vi "Periodic Tasks[Conflict].vi"(8 "error in":errorcluster) -> ()   [LabVIEW 2019]
doc: "This VI runs in parallel to other tasks. It can contain as many user-defined periodic loops as you need. These can carry out PID or other sorts of timed response."
uses:
  <vilib>/Rock Robotics/WPI/ThirdParty/Phoenix-LabVIEW/Motor Controller/Controls/CTRE_Phoenix_MotorControl_ControlMode.ctl
  <vilib>/Rock Robotics/Network Tables/NT Read Number.vi
  <vilib>/Rock Robotics/WPI/ThirdParty/Phoenix-LabVIEW/Motor Controller/Get/CTRE_Phoenix_MotorController_GetSupplyAndStatorCurrent_Enhanced.vi
  <vilib>/Rock Robotics/WPI/ThirdParty/Phoenix-LabVIEW/Motor Controller/Get/CTRE_Phoenix_MotorController_GetSelectedSensorData.vi
  <vilib>/gmath/NI_Gmath.lvlib
panel:
  out "element":dbl
  in  "PIDF?":bool
  in  "Target RPM":dbl
  out "Rpm":cluster{dbl, "Target RPM":dbl}(graph)
  out "Current":T1(graph)
  in  "PIDF Slot":i32
  in  "I-Zone":dbl
  in  "F":dbl=0.055
  in  "D":dbl
  in  "I":dbl
  in  "P":dbl
  out "Target Dist":dbl
  out "Outtake Sensor":bool
  out "Intake Sensor":bool
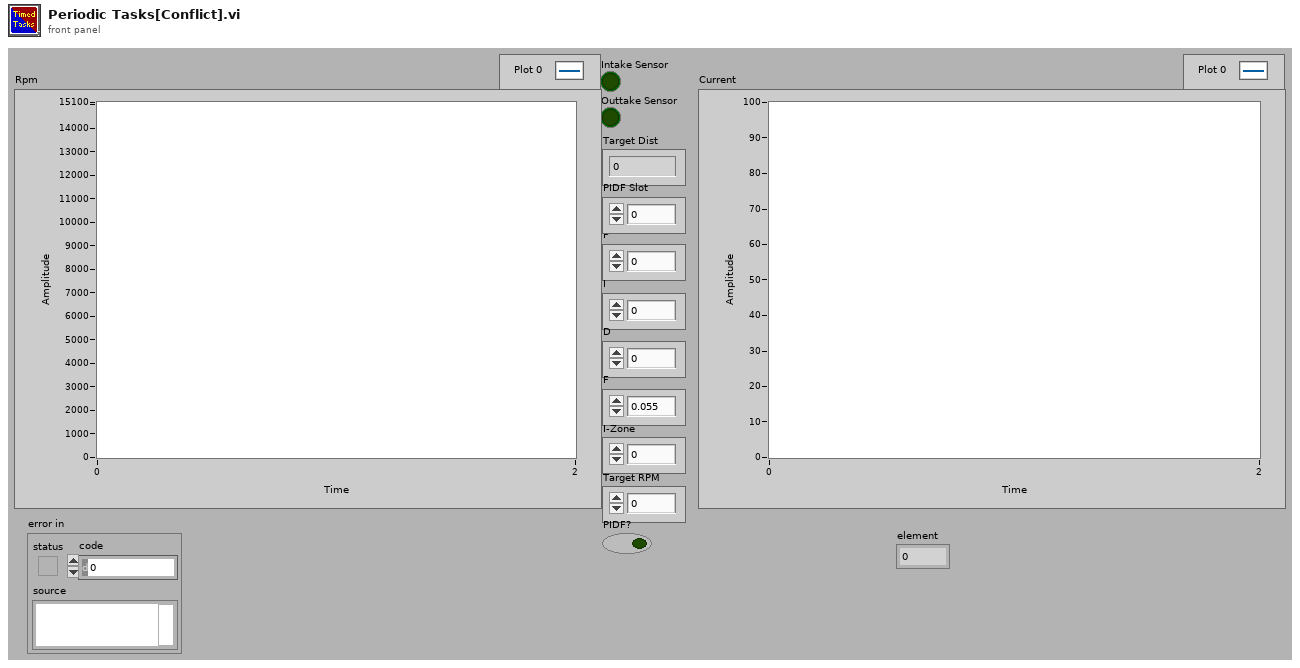
[diagram p1: front panel]
types:
  T1 = cluster{"Supply Current":dbl, "Stator Current":dbl}
  T2 = typedef "WPI_MotorControlDeviceRef.ctl" = cluster{"DeviceStatus":errorcluster, "Type":T3, "PWM":cluster{"PWM Channel":T4, "DeadBand":T5}, "CAN":cluster{"Device Number":u8, "SetOutput VI Ref":variant, "GetOutput VI Ref":variant, "Enable VI Ref":variant, "Disable VI Ref":variant, "Data":variant}, "Invert":bool, "DIO PWM":cluster{"PWM \"Enable\" Channel":T4, "DIOChannel":T6, "PWM Rate":dbl}}
  T3 = typedef "WPI_MotorControlType.ctl" = enum16{"PWM", "CAN", "DIO PWM"}
  T4 = typedef "FPGA_DIOPWMChannel.ctl" = enum8{"PWM 0", "PWM 1", "PWM 2", "PWM 3", "PWM 4", "PWM 5", "PWM 6", "PWM 7", "PWM 8", "PWM 9", "PWM MXP 0", "PWM MXP 1", "PWM MXP 2", "PWM MXP 3", "PWM MXP 4", "PWM MXP 5", "PWM MXP 6", "PWM MXP 7", "PWM MXP 8", "PWM MXP 9", "Invalid"}
  T5 = typedef "WPI_PWMDeadband.ctl" = cluster{"Name":string, "maxPositivePwm":i32, "minPositivePwm":i32, "centerPwm":i32, "maxNegativePwm":i32, "minNegativePwm":i32, "angularRange":u16}
  T6 = typedef "FPGA_DIOChannel.ctl" = enum8{"DIO 0", "DIO 1", "DIO 2", "DIO 3", "DIO 4", "DIO 5", "DIO 6", "DIO 7", "DIO 8", "DIO 9", "DIO MXP 0", "DIO MXP 1", "DIO MXP 2", "DIO MXP 3", "DIO MXP 4", "DIO MXP 5", "DIO MXP 6", "DIO MXP 7", "DIO MXP 8", "DIO MXP 9", "DIO MXP 10", "DIO MXP 11", "DIO MXP 12", "DIO MXP 13", "DIO MXP 14", "DIO MXP 15", "SPI Port CS1", "SPI Port CS2", "SPI Port CS3", "SPI Port MISO", "SPI Port MOSI", "Invalid"}
  T7 = typedef "CTRE_Phoenix_MotorControl_ControlMode.ctl" = u16
  T8 = typedef "WPI_DigitalInputDevRef.ctl" = cluster{"DevStatus":errorcluster, "DIO Channel":T6}
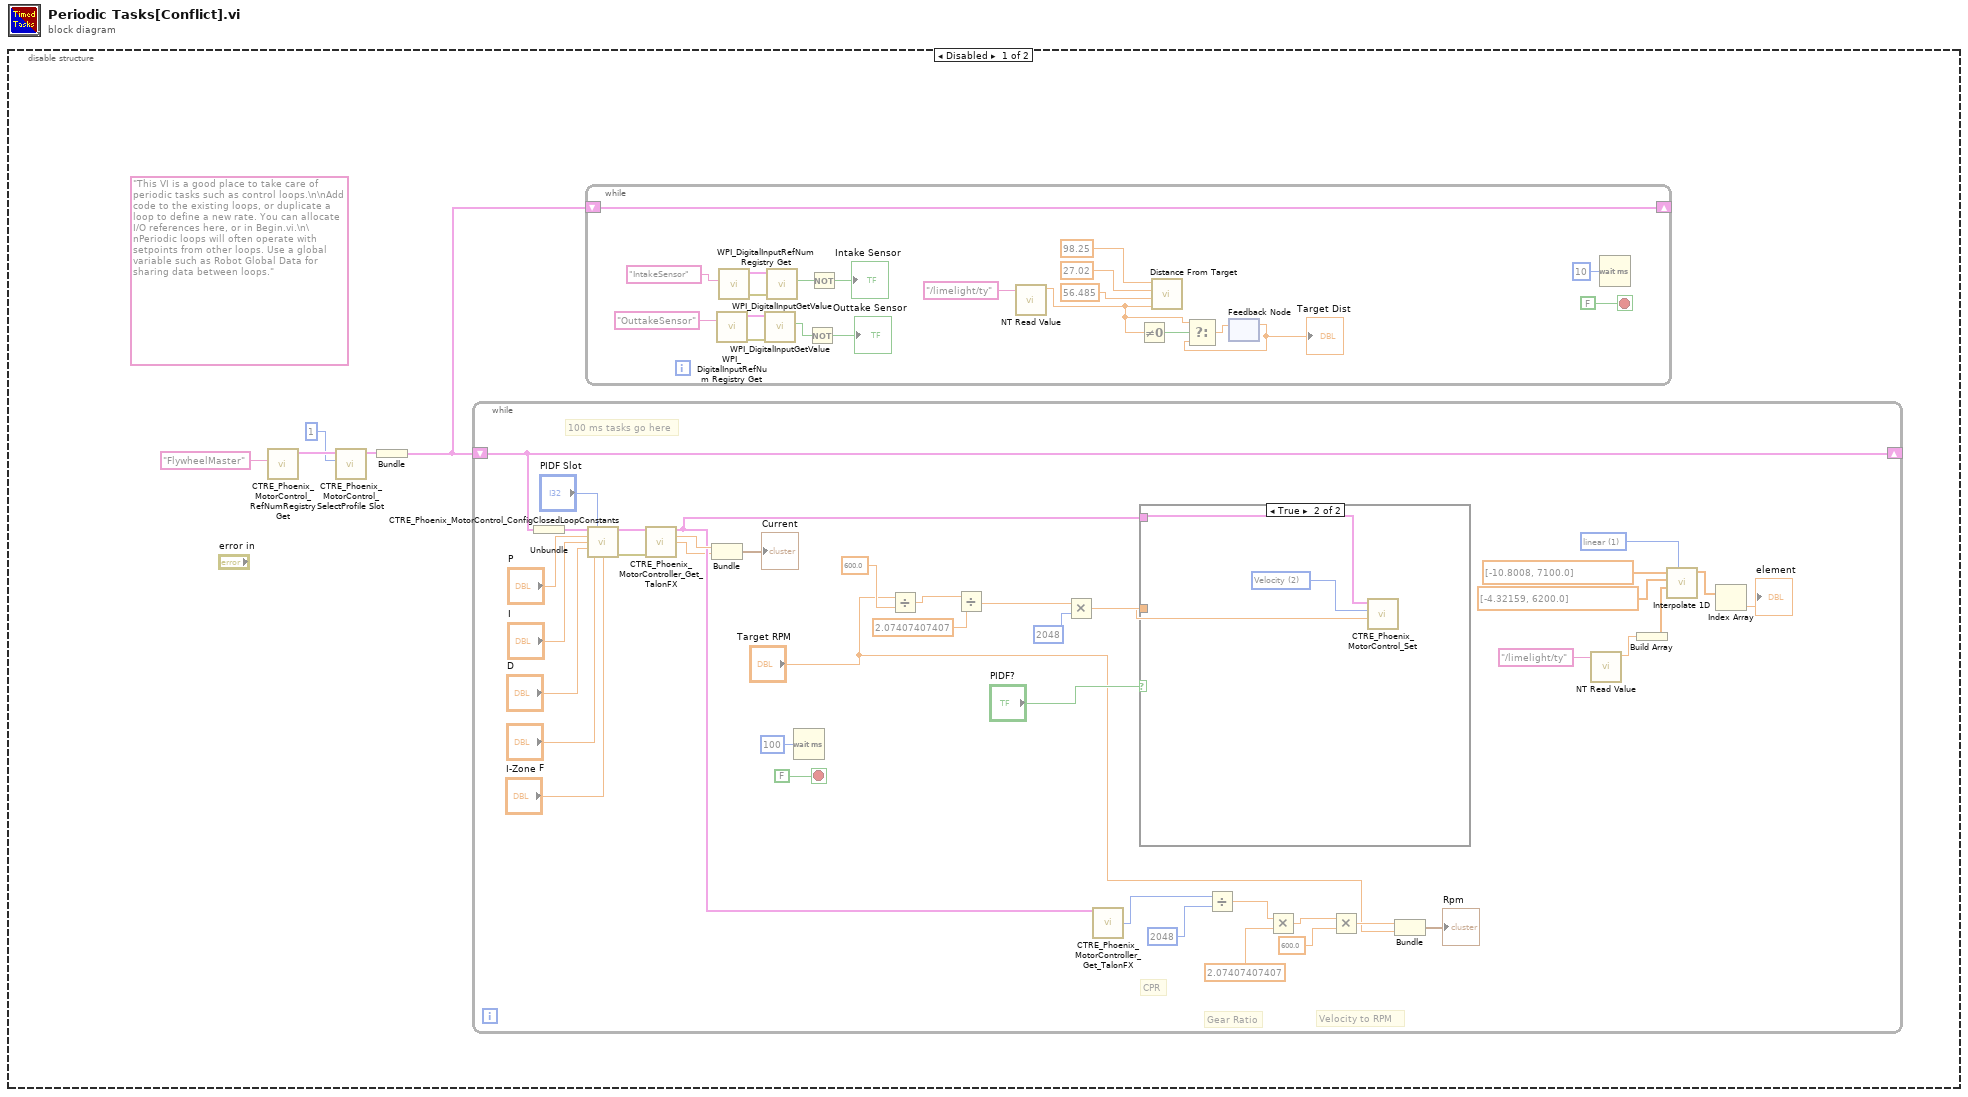
[diagram p0: block diagram]
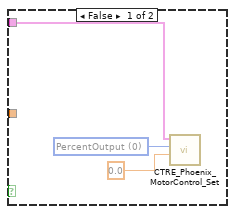
[diagram p2: hidden frame]
diagram:
  n1 = disable-structure shown="Disabled" {
    frame Disabled {
      (unwired) "This VI is a good place to take care of periodic tasks such as control loops.\n\nAdd code to the existing loops, or duplicate a loop to define a new rate. You can allocate I/O references here, or in Begin.vi.\n\nPeriodic loops will often operate with setpoints from other loops. Use a global variable such as Robot Global Data for sharing data between loops."
      n2 = call <vilib>:"CTRE_Phoenix_MotorControl_RefNumRegistryGet.vi"("refnum name"="FlywheelMaster") -> ("PhoenixMotorControlDevRef"=w3:T2)  [unwired: 9 in, 1 out]
      n3 = call <vilib>:"CTRE_Phoenix_MotorControl_SelectProfile Slot.vi"("slotIdx"=1, "PhoenixMotorControlDevRef"=w3) -> ("PhoenixMotorControlDevRef"=w2:T2)  [unwired: 8 in, 1 out]
      n4 = Bundle("PhoenixMotorControlDevRef"=w2) -> (w5:cluster{"PhoenixMotorControlDevRef":T2})  [unwired: 1 out]
      n5 = while {
        shift-right: [w43] -> _
        shift-left: w5 -> [w43]
        stop <- FALSE stop-if-true
        w13 = 1 items=["nearest", "linear", "spline", "cubic Hermite", "Lagrange"] ("method")
        # "CPR"
        # "Velocity to RPM"
        # "Gear Ratio"
        # "100 ms tasks go here"
        n6 = Unbundle(w43) -> ("PhoenixMotorControlDevRef"=w42:T2)
        n7 = call <vilib>:"CTRE_Phoenix_MotorControl_ConfigClosedLoopConstants.vi"("PhoenixMotorControlDevRef"=w42, "slotIdx"="PIDF Slot", "P"="P", "I"="I", "D"="D", "F"="F", "I Zone"="I-Zone") -> ("PhoenixMotorControlDevRef"=w35:T2, "error out"=w34:errorcluster)  [unwired: 7 in]
        n8 = call-poly <vilib>:"CTRE_Phoenix_MotorController_Get_TalonFX.vi"("PhoenixMotorControlDevRef"=w35, "error in"=w34) -> ("PhoenixMotorControlDevRef"=w31:T2, "Supply Current"=w32:dbl, "Stator Current"=w30:dbl)  [unwired: 10 in, 1 out]
        n9 = Bundle("Supply Current"=w32, "Stator Current"=w30) -> (→"Current":T1)  [unwired: 1 out]
        n10 = Wait (ms)(milliseconds to wait=u32 100) -> ()  [unwired: 1 out]
        n11 = Divide(x="Target RPM", y=600.0) -> (x/y=w19:dbl)
        n12 = Divide(x=w19, y=2.07407407407) -> (x/y=w20:dbl)
        n13 = Multiply(x=w20, y=2048) -> (x*y=w15:dbl)
        n14 = call-poly <vilib>:"CTRE_Phoenix_MotorController_Get_TalonFX.vi"("PhoenixMotorControlDevRef"=w31) -> ("Velocity (Raw Sensor Units per 100 ms)"=w25:i32)  [unwired: 11 in, 3 out]
        n15 = case shown="True" "PIDF?" {
          tunnel: w31 -> [w46 w50]
          tunnel: w15 -> [_ w49]
          frame False {
            w47 = T7 0 items=["PercentOutput"=0, "Position"=1, "Velocity"=2, "Current"=3, "Follower"=5, "MotionProfile"=6, "MotionMagic"=7, "MotionProfileArc"=10, "Disabled"=15] ("Control Mode")
            n16 = call <vilib>:"CTRE_Phoenix_MotorControl_Set.vi"("Output"=0.0, "Control Mode"=w47, "PhoenixMotorControlDevRef"=w46) -> ()  [unwired: 7 in, 2 out]
          }
          frame True {
            w51 = T7 2 items=["PercentOutput"=0, "Position"=1, "Velocity"=2, "Current"=3, "Follower"=5, "MotionProfile"=6, "MotionMagic"=7, "MotionProfileArc"=10, "Disabled"=15] ("Control Mode")
            n17 = call <vilib>:"CTRE_Phoenix_MotorControl_Set.vi"("Output"=w49, "Control Mode"=w51, "PhoenixMotorControlDevRef"=w50) -> ()  [unwired: 7 in, 2 out]
          }
        }
        n18 = Divide(x=w25, y=2048) -> (x/y=w24:dbl)
        n19 = Multiply(x=w24, y=2.07407407407) -> (x*y=w26:dbl)
        n20 = Multiply(x=w26, y=600.0) -> (x*y=w27:dbl)
        n21 = Bundle(w27, "Target RPM"="Target RPM") -> (→"Rpm":cluster{dbl, "Target RPM":dbl})  [unwired: 1 out]
        n22 = call-poly <vilib>:"NT Read Value.vi"("Name"="/limelight/ty") -> ("Numeric"=w11:dbl)  [unwired: 9 in, 1 out]
        n23 = Build Array(w11) -> (w10:dbl[])
        n24 = call <vilib>:"Interpolate 1D.vi"("method"=w13, "xi"=w10, "X"=dbl[] [-4.32159, 6200.0] ("Y"), "Y"=dbl[] [-10.8008, 7100.0] ("X")) -> ("yi"=w9:dbl[])  [unwired: 5 in, 2 out]
        n25 = Index Array(array=w9) -> (element=→"element":dbl)  [unwired: 1 in]
      }
      n26 = while {
        shift-right: [w56] -> _
        shift-left: w5 -> [w56]
        stop <- FALSE stop-if-true
        n27 = call <vilib>:"WPI_DigitalInputRefNum Registry Get.vi"("refnum name"="OuttakeSensor") -> ("error out"=w67:errorcluster, "DigitalInputDevRef"=w68:T8)  [unwired: 9 in]
        n28 = call <vilib>:"WPI_DigitalInputRefNum Registry Get.vi"("refnum name"="IntakeSensor") -> ("error out"=w70:errorcluster, "DigitalInputDevRef"=w69:T8)  [unwired: 9 in]
        n29 = call <vilib>:"WPI_DigitalInputGetValue.vi"("error in (no error)"=w67, "DigitalInputDevRef"=w68) -> ("Value"=w65:bool)  [unwired: 7 in, 2 out]
        n30 = call <vilib>:"WPI_DigitalInputGetValue.vi"("error in (no error)"=w70, "DigitalInputDevRef"=w69) -> ("Value"=w66:bool)  [unwired: 7 in, 2 out]
        n31 = Not(x=w65) -> (.not. x?=→"Outtake Sensor":bool)
        n32 = Not(x=w66) -> (.not. x?=→"Intake Sensor":bool)
        n33 = call-poly <vilib>:"NT Read Value.vi"("Name"="/limelight/ty") -> ("Numeric"=w53:dbl)  [unwired: 9 in, 1 out]
        n34 = Not Equal To 0?(x=w53) -> (x != 0?=w55:bool)
        n35 = call "Distance From Target.vi"("Target Angle (Deg)"=w53, "Camera Angle (Deg)"=56.485 ("Camera Angle"), "Camera Height (in)"=27.02, "Target Height (in)"=98.25 ("Camera Height (in)")) -> ()  [unwired: 1 out]
        n36 = feedback #1() -> (w52:dbl)  [unwired: 1 in]
        "Target Dist" <- w52
        n37 = Select(t=w53, s=w55, f=w52) -> (s? t:f=w54:dbl)
        n38 = feedback-in #1(w54) -> ()
        n39 = Wait (ms)(milliseconds to wait=u32 10) -> ()  [unwired: 1 out]
      }
    }
    frame Enabled {
    }
  }
